vi "CUMain.vi"() -> ()   [LabVIEW 2013]
doc: "Use this template to build a simple state machine design pattern. Each state executes code and determines which state to transition to."
uses:
  controls/CUState.ctl
  controls/CUData.ctl
  <vilib>/Instr/_visa.llb/VISA Configure Serial Port (Instr).vi
panel:
  in  "Send A-V command":bool
  in  "Value (U16)":u16 format="%04x"
  in  "Address (U16)":u16=255 format="%04x"
  in  "Keep send encode string":bool
  in  "Enable read":bool=TRUE
  out "Read string":string
  in  "Bytes to read":u32=512
  out "Actual bytes read":u32
  in  "Clear text":bool
  out "Encoded string":string
  in  "Send string":string="DA1 0C1 <<< SM1 SM2 SM3 >>> MM1"
  in  "stop bits":u16(ring)=10 items=["1.0"=10, "1.5"=15, "2.0"=20]
  in  "parity":u16(ring) items=["None", "Odd", "Even", "Mark", "Space"]
  in  "data bits":u16=8 min=5 max=8 step=1
  in  "VISA resource name":refnum<visa-resource-name>="COM1"
  in  "baud rate":u32=9600
  in  "Send ASCII command":bool
  in  "Stop Button":bool
  # "(Add SPACE between ASCII commands)"
  # "(Press ENTER to send when value ready)"
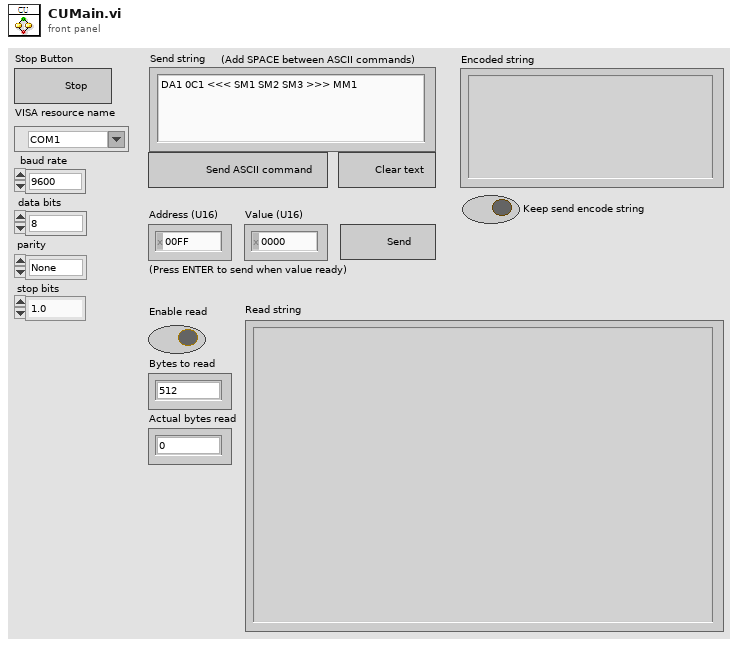
[diagram p1: front panel]
types:
  T1 = typedef "CUData.ctl" = cluster{"String to send":string, "Encoded string to send":string}
  T2 = typedef "CUState.ctl" = enum16{"Initialize", "Wait for Event", "Encode ASCII command", "Encode A-V command", "Send command", "Read data", "Stop"}
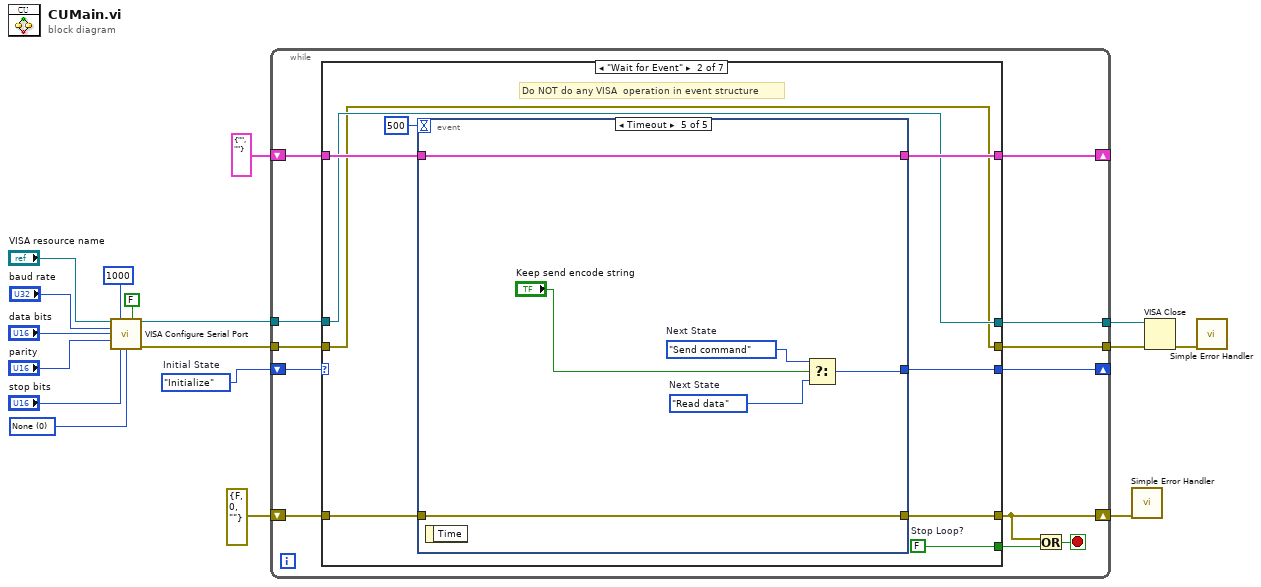
[diagram p0: block diagram]
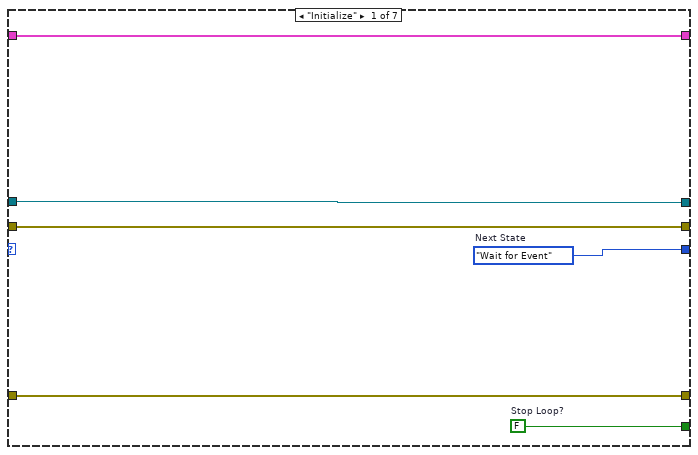
[diagram p2: hidden frame]
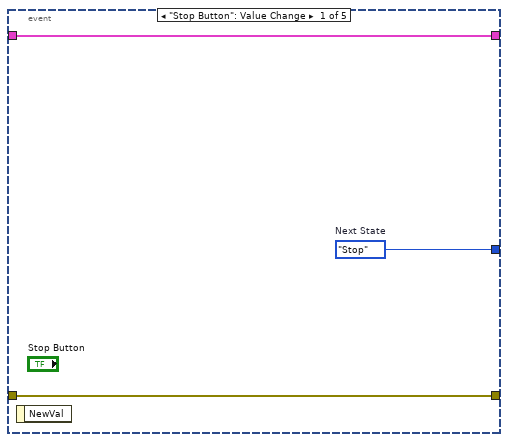
[diagram p3: hidden frame]
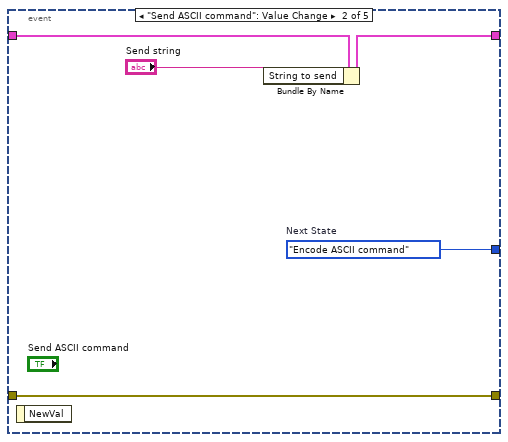
[diagram p4: hidden frame]
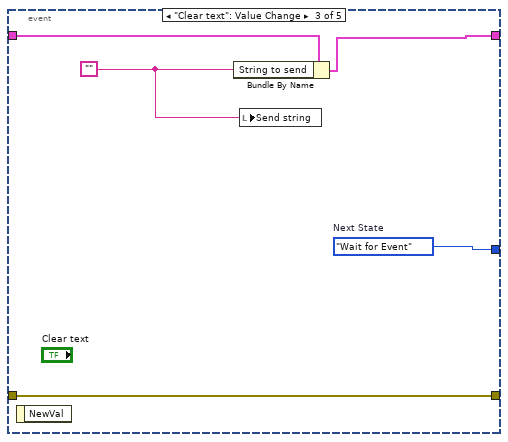
[diagram p5: hidden frame]
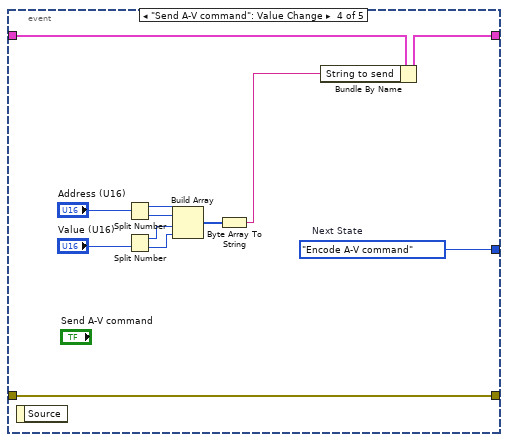
[diagram p6: hidden frame]
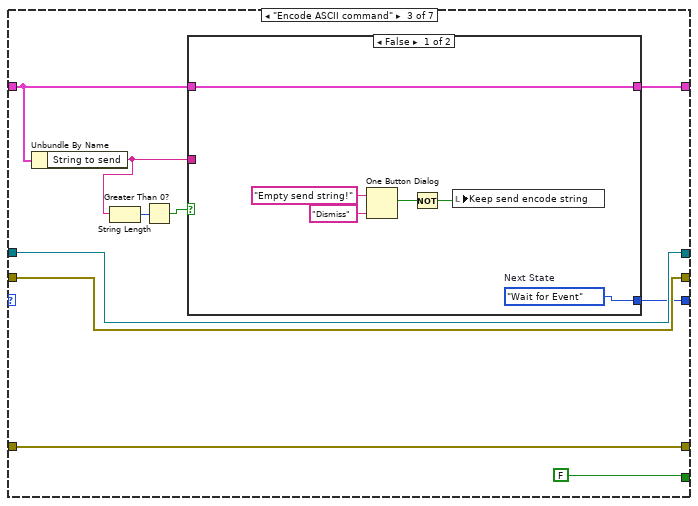
[diagram p7: hidden frame]
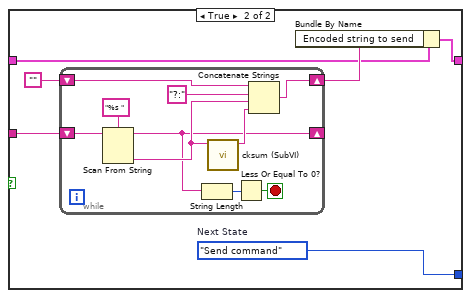
[diagram p8: hidden frame]
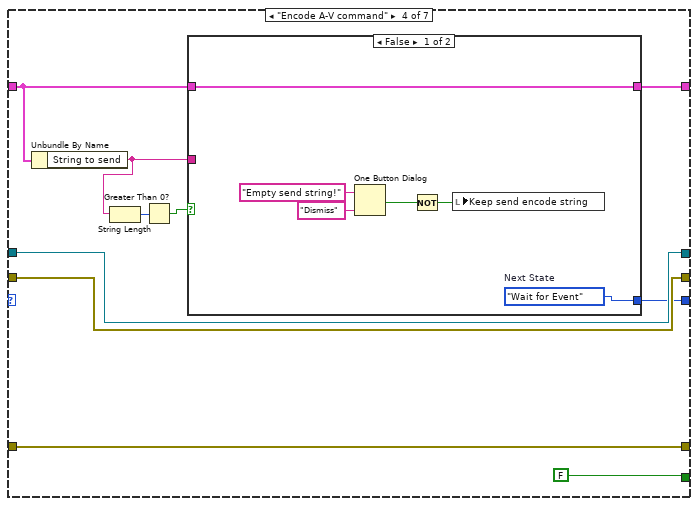
[diagram p9: hidden frame]
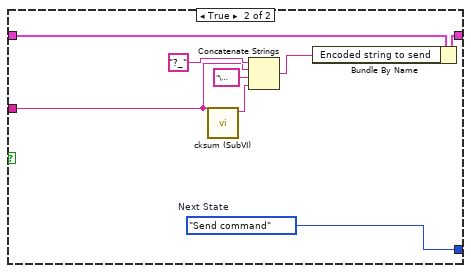
[diagram p10: hidden frame]
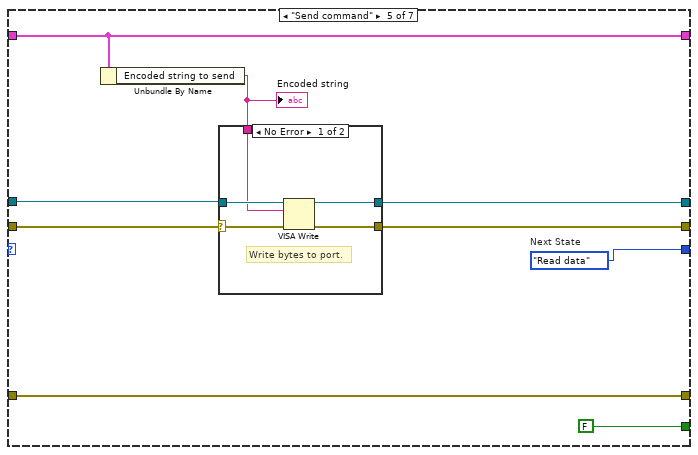
[diagram p11: hidden frame]
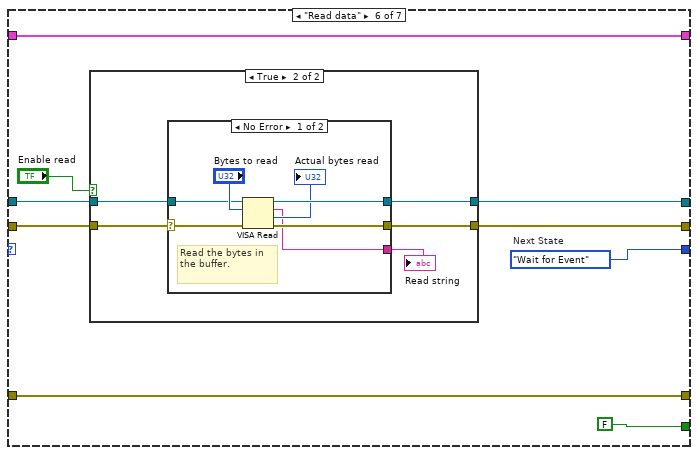
[diagram p13: hidden frame]
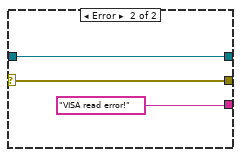
[diagram p15: hidden frame]
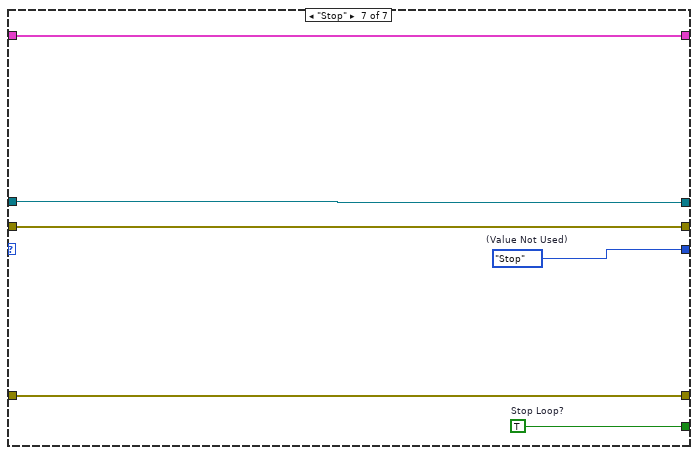
[diagram p16: hidden frame]
diagram:
  w7 = u16 0 items=["None"=0, "XON/XOFF"=1, "RTS/CTS"=2, "DTR/DSR"=4] ("flow control")
  w17 = CUState."Initialize"  # Initial State
  n1 = call-poly "VISA Configure Serial Port"("VISA resource name"="VISA resource name", "timeout (10sec)"=u32 1000 ("timeout (ms)"), "Enable Termination\nChar (T)"=FALSE ("End read on termination character?"), "baud rate (9600)"="baud rate", "data bits (8)"="data bits", "parity (0:none)"="parity", "stop bits (10: 1 bit)"="stop bits", "flow control (0:none)"=w7) -> ("VISA resource name out"=w3:refnum<visa-resource-name>, "error out"=w2:errorcluster)  [unwired: 2 in, 4 out]
  n2 = while {
    shift-right: [w28] -> _
    shift-left: w17 -> [w29]
    shift-right: [w26] -> _
    shift-left: T1 {"String to send"="", "Encoded string to send"=""} ("Data") -> [w27]
    shift-right: [w22] -> w14
    shift-left: errorcluster {"status"=FALSE, "code"=0, "source"=""} ("error constant") -> [w25]
    tunnel: [w21] -> w4
    tunnel: w3 -> [w20]
    tunnel: w2 -> [w19]
    tunnel: [w18] -> w1
    stop <- w23 stop-if-true
    n3 = case shown="\"Wait for Event\"" w29 {
      tunnel: [w35 w44 w82 w114 w140 w148 w179] -> w28
      tunnel: [w34 w43 FALSE ("Stop Loop?") FALSE ("Stop Loop?") FALSE ("Stop Loop?") FALSE ("Stop Loop?") w177] -> w24
      tunnel: w27 -> [w30 w42 w80 w112 w132 w149 w178]
      tunnel: [w30 w41 w79 w111 w132 w149 w178] -> w26
      tunnel: w25 -> [w33 w40 w85 w117 w138 w156 w176]
      tunnel: [w33 w39 w85 w117 w138 w156 w176] -> w22
      tunnel: [w32 w38 w84 w116 w136 w154 w175] -> w21
      tunnel: w20 -> [w32 w38 w84 w116 w137 w155 w175]
      tunnel: w19 -> [w31 w37 w83 w115 w134 w152 w174]
      tunnel: [w31 w37 w83 w115 w135 w153 w174] -> w18
      frame "Initialize" {
        w34 = FALSE  # Stop Loop?
        w35 = CUState."Wait for Event"  # Next State
      }
      frame "Wait for Event" {
        w43 = FALSE  # Stop Loop?
        # "Do NOT do any VISA  operation in event structure"
        n4 = event shown="[4] Timeout" {
          selector: _ -> [_ _ _ _ _]
          dyn-events: _ -> [_ _ _ _ _]
          timeout: 500 -> [_ _ _ _ _]
          tunnel: [w47 w52 w54 w69 w72] -> w44
          tunnel: w42 -> [w46 w51 w56 w68 w74]
          tunnel: [w46 w50 w55 w67 w74] -> w41
          tunnel: w40 -> [w45 w48 w57 w66 w75]
          tunnel: [w45 w48 w57 w66 w75] -> w39
          event "Stop Button": Value Change {
            w47 = CUState."Stop"  # Next State
            n5 = event-data() -> ()  [unwired: 1 in, 1 out]
          }
          event "Send ASCII command": Value Change {
            w52 = CUState."Encode ASCII command"  # Next State
            n6 = event-data() -> ()  [unwired: 1 in, 1 out]
            n7 = Bundle By Name(cluster=w51, "String to send"="Send string") -> (w50:T1)
          }
          event "Clear text": Value Change {
            w54 = CUState."Wait for Event"  # Next State
            w53 = "" ("String to send")
            n8 = event-data() -> ()  [unwired: 1 in, 1 out]
            n9 = Bundle By Name(cluster=w56, "String to send"=w53) -> (w55:T1)
            n10 = local write "Send string"(w53) -> ()
          }
          event "Send A-V command": Value Change {
            w69 = CUState."Encode A-V command"  # Next State
            n11 = event-data() -> ()  [unwired: 1 in, 1 out]
            n12 = Split Number(x="Address (U16)") -> (hi(x)=w63:u8, lo(x)=w62:u8)
            n13 = Split Number(x="Value (U16)") -> (hi(x)=w61:u8, lo(x)=w60:u8)
            n14 = Build Array(w63, w62, w61, w60) -> (w59:u8[])
            n15 = Byte Array To String(unsigned byte array=w59) -> (string=w58:string)
            n16 = Bundle By Name(cluster=w68, "String to send"=w58) -> (w67:T1)
          }
          event Timeout {
            w71 = CUState."Send command"  # Next State
            w70 = CUState."Read data"  # Next State
            n17 = event-data() -> ()  [unwired: 1 in, 1 out]
            n18 = Select(t=w71, s="Keep send encode string", f=w70) -> (s? t:f=w72:T2)
          }
        }
      }
      frame "Encode ASCII command" {
        n19 = Unbundle By Name(w80) -> ("String to send"=w77:string)
        n20 = String Length(string=w77) -> (length=w78:i32)
        n21 = Greater Than 0?(x=w78) -> (x > 0?=w76:bool)
        n22 = case shown="False" w76 {
          tunnel: [w91 w97] -> w82
          tunnel: w77 -> [_ w96]
          tunnel: w80 -> [w89 w94]
          tunnel: [w89 w93] -> w79
          frame False {
            w91 = CUState."Wait for Event"  # Next State
            n23 = One Button Dialog(message="Empty send string!", button name ("OK")="Dismiss") -> (true=w86:bool)
            n24 = Not(x=w86) -> (.not. x?=w87:bool)
            n25 = local write "Keep send encode string"(w87) -> ()
          }
          frame True {
            w97 = CUState."Send command"  # Next State
            n26 = while {
              shift-right: [w100] -> _
              shift-left: w96 -> [w107]
              shift-right: [w103] -> w95
              shift-left: "" -> [w98]
              stop <- w104 stop-if-true
              n27 = Scan From String(format string="%s ", input string=w107) -> (remaining string=w100:string, output 1=w102:string)  [unwired: 3 in, 2 out]
              n28 = String Length(string=w100) -> (length=w105:i32)
              n29 = call "cksum (SubVI).vi"("Input String"=w102) -> ("Checksum"=w101:string)  [unwired: 10 in]
              n30 = Less Or Equal To 0?(x=w105) -> (x <= 0?=w104:bool)
              n31 = Concatenate Strings(w98, "?:", w102, w101) -> (w103:string)
            }
            n32 = Bundle By Name(cluster=w94, "Encoded string to send"=w95) -> (w93:T1)
          }
        }
      }
      frame "Encode A-V command" {
        n33 = Unbundle By Name(w112) -> ("String to send"=w109:string)
        n34 = String Length(string=w109) -> (length=w110:i32)
        n35 = Greater Than 0?(x=w110) -> (x > 0?=w108:bool)
        n36 = case shown="False" w108 {
          tunnel: [w123 w131] -> w114
          tunnel: w109 -> [_ w125]
          tunnel: w112 -> [w121 w129]
          tunnel: [w121 w128] -> w111
          frame False {
            w123 = CUState."Wait for Event"  # Next State
            n37 = One Button Dialog(message="Empty send string!", button name ("OK")="Dismiss") -> (true=w118:bool)
            n38 = Not(x=w118) -> (.not. x?=w119:bool)
            n39 = local write "Keep send encode string"(w119) -> ()
          }
          frame True {
            w131 = CUState."Send command"  # Next State
            n40 = call "cksum (SubVI).vi"("Input String"=w125) -> ("Checksum"=w127:string)  [unwired: 10 in]
            n41 = Concatenate Strings("?_", w125, "\u0000" ("string"), w127) -> (w130:string)
            n42 = Bundle By Name(cluster=w129, "Encoded string to send"=w130) -> (w128:T1)
          }
        }
      }
      frame "Send command" {
        w140 = CUState."Read data"  # Next State
        n43 = Unbundle By Name(w132) -> ("Encoded string to send"=w133:string)
        "Encoded string" <- w133
        n44 = case shown="No Error" w134 {
          selector: w134 -> [w142 w147]
          tunnel: [w145 w146] -> w136
          tunnel: [w144 w147] -> w135
          tunnel: w137 -> [w143 w146]
          tunnel: w133 -> [w141 _]
          frame No Error {
            # "Write bytes to port."
            n45 = VISA Write(VISA resource name=w143, write buffer=w141, error in (no error)=w142) -> (VISA resource name out=w145:refnum<visa-resource-name>, error out=w144:errorcluster)  [unwired: 1 out]
          }
          frame Error {
          }
        }
      }
      frame "Read data" {
        w148 = CUState."Wait for Event"  # Next State
        n46 = case shown="True" "Enable read" {
          tunnel: w155 -> [w158 w163]
          tunnel: [w158 w162] -> w154
          tunnel: [w157 w161] -> w153
          tunnel: w152 -> [w157 w160]
          frame False {
          }
          frame True {
            n47 = case "Read bytes from port." shown="No Error" w160 {
              selector: w160 -> [w166 w172]
              tunnel: [w169 w172] -> w161
              tunnel: [w170 w173] -> w162
              tunnel: w163 -> [w167 w173]
              tunnel: [w164 "VISA read error!" ("read buffer")] -> w159
              frame No Error {
                # "Read the bytes in the buffer."
                n48 = VISA Read(VISA resource name=w167, byte count="Bytes to read", error in (no error)=w166) -> (VISA resource name out=w170:refnum<visa-resource-name>, read buffer=w164:string, return count=→"Actual bytes read":u32, error out=w169:errorcluster)
              }
              frame Error {
                # "Error occurred \nreading Bytes at \nSerial Port"
              }
            }
            "Read string" <- w159
          }
        }
      }
      frame "Stop" {
        w177 = TRUE  # Stop Loop?
        w179 = CUState."Stop"  # (Value Not Used)
      }
    }
    n49 = Or(x=w22, y=w24) -> (x .or. y?=w23:bool)
  }
  n50 = call <vilib>:"Simple Error Handler.vi"("error in (no error)"=w14) -> ()  [unwired: 4 in, 5 out]
  n51 = VISA Close(VISA resource name=w4, error in (no error)=w1) -> (error out=w5:errorcluster)
  n52 = call <vilib>:"Simple Error Handler.vi"("error in (no error)"=w5) -> ()  [unwired: 1 in, 8 out]
